vi "Call Config.vi"(8 "error in (no error)":errorcluster, 10 "Command":string) -> (0 "error out":errorcluster)   [LabVIEW 2018, in "Configuration.lvlib"]
uses:
  Configuration.lvlib
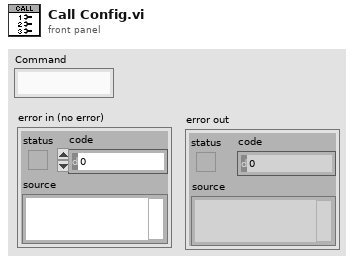
[diagram p1: front panel]
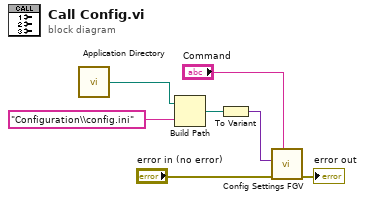
[diagram p0: block diagram]
diagram:
  n1 = call <vilib>:"Application Directory.vi"() -> ("Application Directory"=w4:path)
  n2 = Build Path(base path=w4, name or relative path="Configuration\\config.ini") -> (appended path=w6:path)
  n3 = To Variant(anything=w6) -> (Variant=w7:variant)
  n4 = call "Config Settings FGV.vi"("Command"="Command", "error in (no error)"="error in (no error)", "Data in"=w7) -> ("error out"=→"error out":errorcluster)  [unwired: 7 in, 1 out]
